vi "Camera_Focusing.vi"(8 "CURRENT MEAN VALUE":refnum<vi>, 9 "Filter Type":T2(ring)=enum."Differentiation", 10 "MEAN VALUE MAX":refnum<vi>, 11 "Image Path":path=path "C:/images/img1.jpeg") -> (0 "error out":errorcluster, 1 "Curent Mean Value":sgl=4.1535125 format="%.2f", 2 "Mean Value Max":sgl=4.1535125 format="%.2f", 3 "Pattern Presence":bool=TRUE, 4 "Reverse":bool, 5 "Image out":T1(plugin-control))   [LabVIEW 2018]
uses:
  <vilib>/vision/NI_Vision_Development_Module.lvlib
panel:
  in  "error in":errorcluster
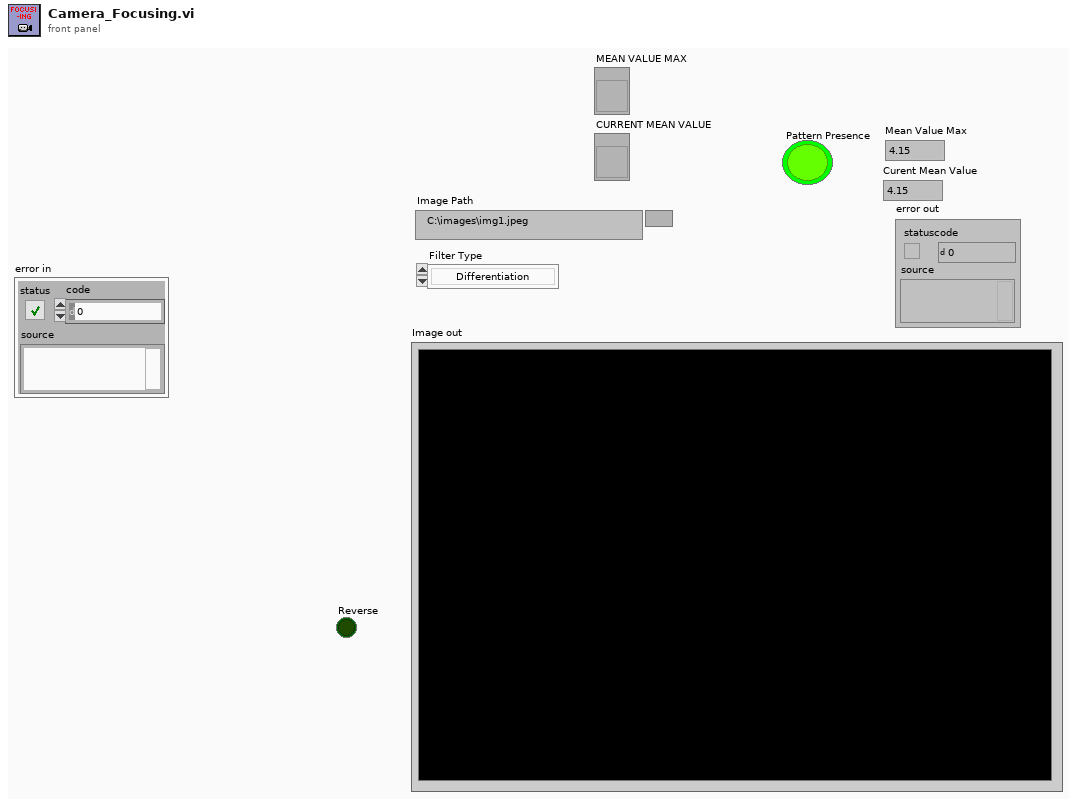
[diagram p1: front panel]
types:
  T1 = typedef "IMAQ Image.ctl" = refnum<image>
  T2 = enum16{"Convolution", "Differentiation", "Gradient", "Prewitt", "Roberts", "Sigma", "Sobel"}
  T3 = enum32{"Differentiation", "Gradient", "Prewitt", "Roberts", "Sigma", "Sobel"}
  T4 = typedef "Image Type" = u32
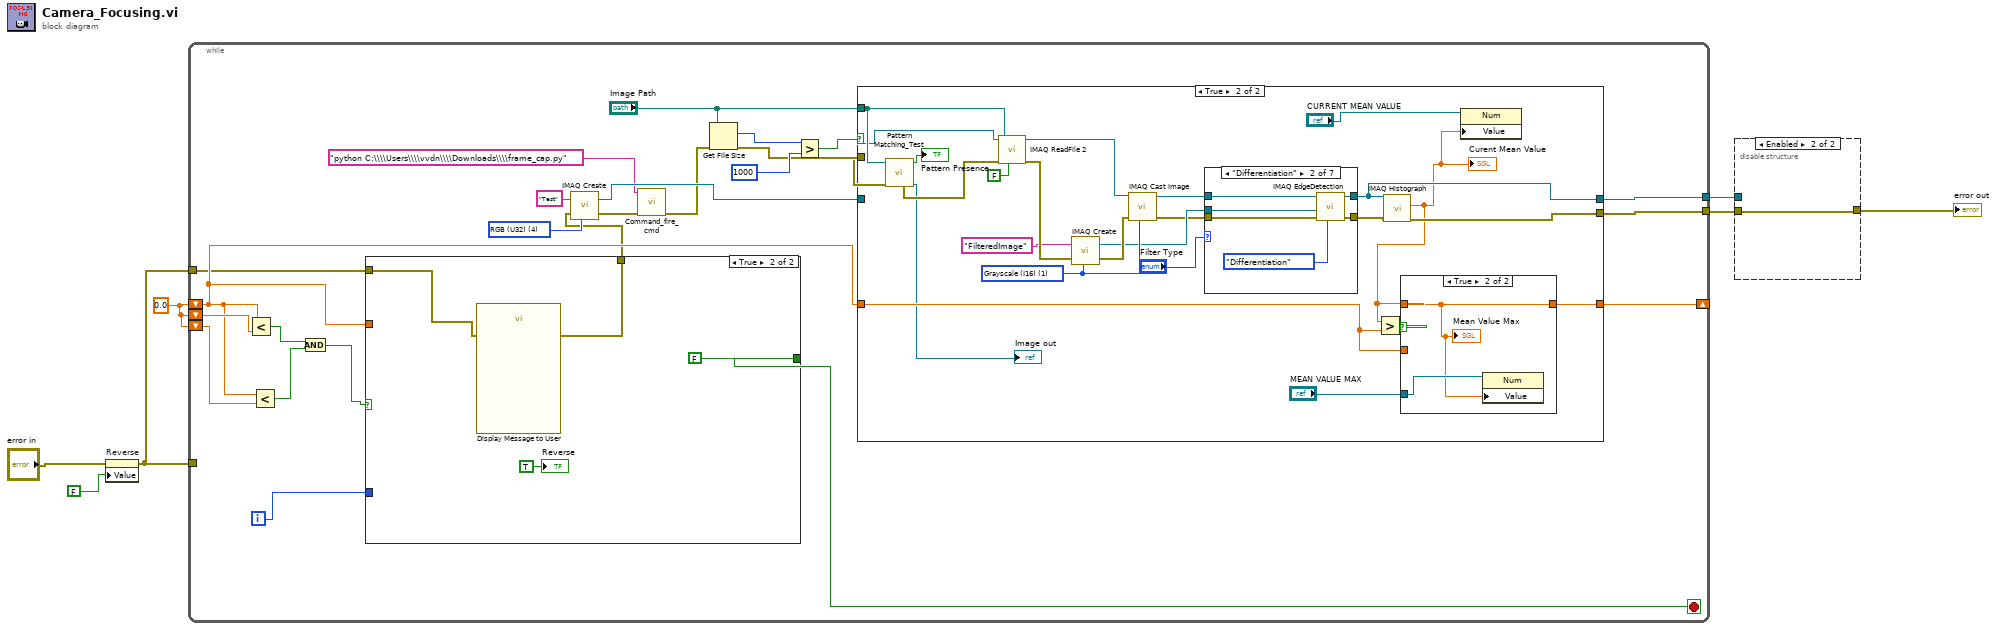
[diagram p0: block diagram]
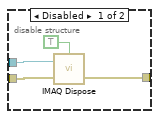
[diagram p2: hidden frame]
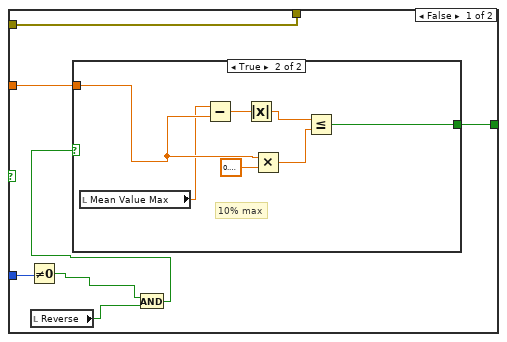
[diagram p3: hidden frame]
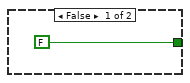
[diagram p4: hidden frame]
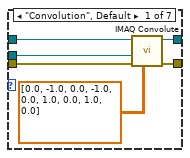
[diagram p7: hidden frame]
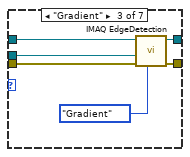
[diagram p8: hidden frame]
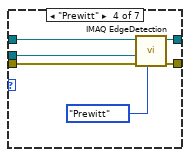
[diagram p9: hidden frame]
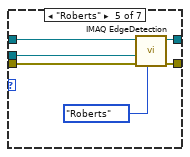
[diagram p10: hidden frame]
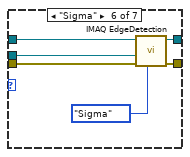
[diagram p11: hidden frame]
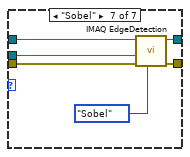
[diagram p12: hidden frame]
diagram:
  w1 = 0.0
  n1 = property on="Reverse" class="Bool"(error in="error in", "Value"=FALSE ("Reverse")) -> (error out=w2:errorcluster)  [unwired: 1 in, 1 out]
  n2 = while {
    tunnel: [w31] -> w7
    tunnel: [w30] -> w6
    shift-right: [w19] -> _
    shift-left: w1 -> [w13]
    shift-left: w1 -> [w16]
    shift-left: w1 -> [w15]
    tunnel: w2 -> [w10]
    tunnel: w2 -> [_]
    i -> [w14]
    stop <- w12 stop-if-true
    w28 = T4 4 items=["Grayscale (U8)", "Grayscale (I16)", "Grayscale (SGL)", "Complex (CSG)", "RGB (U32)", "HSL (U32)", "RGB (U64)", "Grayscale (U16)"] ("Image Type")
    n3 = Less?(x=w13, y=w16) -> (x < y?=w18:bool)
    n4 = Less?(x=w13, y=w15) -> (x < y?=w17:bool)
    n5 = And(x=w18, y=w17) -> (x .and. y?=w9:bool)
    n6 = case shown="True" w9 {
      tunnel: w14 -> [w37 _]
      tunnel: [w38 FALSE] -> w12
      tunnel: w13 -> [w36 _]
      tunnel: [w32 w48] -> w11
      tunnel: w10 -> [w32 w47]
      frame False {
        n7 = Not Equal To 0?(x=w37) -> (x != 0?=w34:bool)
        n8 = local read "Reverse"() -> (w35:bool)
        n9 = And(x=w34, y=w35) -> (x .and. y?=w33:bool)
        n10 = case shown="True" w33 {
          tunnel: [FALSE w44] -> w38
          tunnel: w36 -> [_ w41]
          frame False {
          }
          frame True {
            # "10% max"
            n11 = local read "Mean Value Max"() -> (w40:sgl)
            n12 = Subtract(x=w40, y=w41) -> (x-y=w46:dbl)
            n13 = Absolute Value(x=w46) -> (abs(x)=w42:dbl)
            n14 = Multiply(x=w41, y=sgl 0.1) -> (x*y=w43:dbl)
            n15 = Less Or Equal?(x=w42, y=w43) -> (x <= y?=w44:bool)
          }
        }
      }
      frame True {
        n16 = call "Display Message to User"("error in (no error)"=w47) -> ("error out"=w48:errorcluster)  [unwired: 9 in, 1 out]
        "Reverse" <- TRUE ("Reverse")
      }
    }
    n17 = call "IMAQ Create"("Image Name"="Test", "Image Type"=w28, "error in (no error)"=w11) -> ("New Image"=w22:T1, "error out"=w23:errorcluster)  [unwired: 2 in]
    n18 = call "Command_fire_cmd.vi"("error in"=w23, "command line"="python C:\\\\Users\\\\vvdn\\\\Downloads\\\\frame_cap.py") -> ("error out"=w21:errorcluster)  [unwired: 5 in, 2 out]
    n19 = Get File Size(file="Image Path", error in=w21) -> (size (in bytes)=w26:i64, 0:w20:errorcluster)  [unwired: 1 out]
    n20 = Greater?(x=w26, y=i64 1000) -> (0:w24:bool)
    n21 = case shown="True" w24 {
      tunnel: "Image Path" -> [_ w77]
      tunnel: w20 -> [w52 w76]
      tunnel: [w53 w63] -> w19
      tunnel: w13 -> [w53 w59]
      tunnel: w22 -> [w51 w62]
      tunnel: [w52 w61] -> w31
      tunnel: [w51 w60] -> w30
      frame False {
      }
      frame True {
        w70 = T4 1 items=["Grayscale (U8)", "Grayscale (I16)", "Grayscale (SGL)", "Complex (CSG)", "RGB (U32)", "HSL (U32)", "RGB (U64)", "Grayscale (U16)"] ("Image Type")
        n22 = call "Pattern Matching_Test.vi"("error in (no error)"=w76, "File Path"=w77) -> ("Image out"=→"Image out":T1, "Pattern Presence"=→"Pattern Presence":bool, "error out"=w75:errorcluster)  [unwired: 5 in, 2 out]
        n23 = call "IMAQ ReadFile 2"("Use File Path Image Type"=FALSE, "File Path"=w77, "error in (no error)"=w75, "Image"=w62) -> ("error out"=w73:errorcluster, "Image Out"=w58:T1)  [unwired: 3 in, 3 out]
        n24 = call "IMAQ Create"("Image Name"="FilteredImage", "Image Type"=w70, "error in (no error)"=w73) -> ("New Image"=w67:T1, "error out"=w71:errorcluster)  [unwired: 2 in]
        n25 = call "IMAQ Cast Image"("Image Type"=w70, "error in (no error)"=w71, "Image Src"=w58) -> ("error out"=w66:errorcluster, "Image Dst Out"=w68:T1)  [unwired: 7 in]
        n26 = case shown="\"Differentiation\"" "Filter Type" {
          tunnel: w68 -> [w86 w92 w98 w104 w110 w116 w122]
          tunnel: w66 -> [w85 w91 w97 w103 w109 w115 w121]
          tunnel: w67 -> [w84 w93 w99 w105 w111 w117 w123]
          tunnel: [w83 w88 w94 w100 w106 w112 w118] -> w65
          tunnel: [w82 w89 w95 w101 w107 w113 w119] -> w60
          frame "Convolution", Default {
            n27 = call "IMAQ Convolute"("Kernel"=sgl[][] [[0.0, -1.0, 0.0], [-1.0, 0.0, 1.0], [0.0, 1.0, 0.0]], "error in (no error)"=w85, "Image Dst"=w84, "Image Src"=w86) -> ("error out"=w83:errorcluster, "Image Dst Out"=w82:T1)  [unwired: 6 in]
          }
          frame "Differentiation" {
            n28 = call "IMAQ EdgeDetection"("Method"=T3."Differentiation", "error in (no error)"=w91, "Image Dst"=w93, "Image Src"=w92) -> ("error out"=w88:errorcluster, "Image Dst Out"=w89:T1)  [unwired: 6 in]
          }
          frame "Gradient" {
            n29 = call "IMAQ EdgeDetection"("Method"=T3."Gradient", "error in (no error)"=w97, "Image Dst"=w99, "Image Src"=w98) -> ("error out"=w94:errorcluster, "Image Dst Out"=w95:T1)  [unwired: 6 in]
          }
          frame "Prewitt" {
            n30 = call "IMAQ EdgeDetection"("Method"=T3."Prewitt", "error in (no error)"=w103, "Image Dst"=w105, "Image Src"=w104) -> ("error out"=w100:errorcluster, "Image Dst Out"=w101:T1)  [unwired: 6 in]
          }
          frame "Roberts" {
            n31 = call "IMAQ EdgeDetection"("Method"=T3."Roberts", "error in (no error)"=w109, "Image Dst"=w111, "Image Src"=w110) -> ("error out"=w106:errorcluster, "Image Dst Out"=w107:T1)  [unwired: 6 in]
          }
          frame "Sigma" {
            n32 = call "IMAQ EdgeDetection"("Method"=T3."Sigma", "error in (no error)"=w115, "Image Dst"=w117, "Image Src"=w116) -> ("error out"=w112:errorcluster, "Image Dst Out"=w113:T1)  [unwired: 6 in]
          }
          frame "Sobel" {
            n33 = call "IMAQ EdgeDetection"("Method"=T3."Sobel", "error in (no error)"=w121, "Image Dst"=w123, "Image Src"=w122) -> ("error out"=w118:errorcluster, "Image Dst Out"=w119:T1)  [unwired: 6 in]
          }
        }
        n34 = call "IMAQ Histograph"("error in (no error)"=w65, "Image"=w60) -> ("error out"=w61:errorcluster, "Mean Value"=w54:sgl)  [unwired: 6 in, 2 out]
        "Curent Mean Value" <- w54
        n35 = Greater?(x=w54, y=w59) -> (0:w64:bool)
        n36 = case shown="True" w64 {
          tunnel: w54 -> [_ w80]
          tunnel: [w79 w80] -> w63
          tunnel: w59 -> [w79 _]
          tunnel: "MEAN VALUE MAX" -> [_ w81]
          frame False {
          }
          frame True {
            n37 = property class="Num"(reference=w81, "Value"=w80) -> ()  [unwired: 1 in, 2 out]
            "Mean Value Max" <- w80
          }
        }
        n38 = property class="Num"(reference="CURRENT MEAN VALUE", "Value"=w54) -> ()  [unwired: 1 in, 2 out]
      }
    }
  }
  n39 = disable-structure shown="Enabled" {
    disable-tunnel: w7 -> [w127 w128]
    disable-tunnel: w6 -> [w126 _]
    disable-tunnel: [w124 w128] -> w5
    frame Disabled {
      n40 = call "IMAQ Dispose"("All Images? (No)"=TRUE, "Image"=w126, "error in (no error)"=w127) -> ("error out"=w124:errorcluster)  [unwired: 3 in]
    }
    frame Enabled {
    }
  }
  "error out" <- w5
